vi "Add Virtual Instrument.vi"(8 "Error In":errorcluster, 9 "IVirtual Instrument":refnum<class "IVirtual Instrument.lvclass">, 10 "Instrument Identifier":string) -> (0 "Error Out":errorcluster)   [LabVIEW 2019, in "Instrument Manager.lvclass"]
uses:
  Instrument Manager.lvclass
  Instrument Manager.lvclass/Instrument Manager.ctl
  Interfaces/IVirtual Instrument/IVirtual Instrument.lvclass
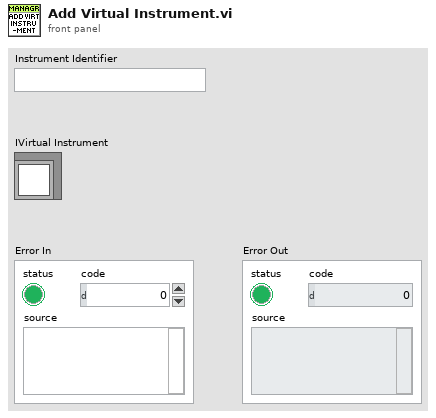
[diagram p1: front panel]
types:
  T1 = typedef "Instrument Manager.lvclass/ObjectAttributes.ctl" = cluster{"ICreate Action Point":refnum<class "ICreate Action Point.lvclass">, "IInstruments":map{string, refnum<class "IInstrument.lvclass">}, "IVirtual Instruments":map{string, refnum<class "IVirtual Instrument.lvclass">}, "Instrument Configurations":map{string, refnum<class "Config from JSON.lvclass">}, "Virtual Instrument Configurations":map{string, refnum<class "Config from JSON.lvclass">}, "Action Point Configurations":map{string, refnum<class "Config from JSON.lvclass">}, "Action Points":map{string, refnum<class "Action Point.lvclass">}}
  T2 = map{string, refnum<class "IVirtual Instrument.lvclass">}
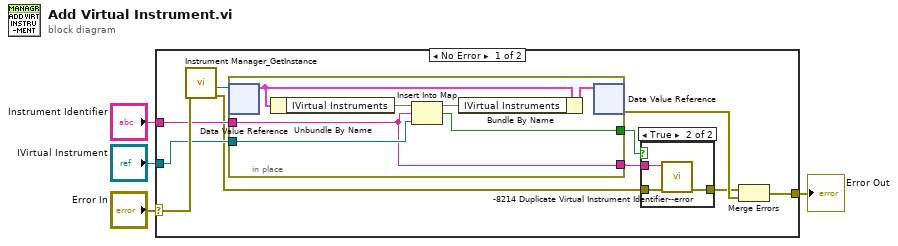
[diagram p0: block diagram]
diagram:
  n1 = case shown="No Error" "Error In" {
    selector: "Error In" -> [w14 w26]
    tunnel: [w12 w26] -> w3
    tunnel: "IVirtual Instrument" -> [w10 _]
    tunnel: "Instrument Identifier" -> [w9 _]
    frame No Error {
      n2 = call "Instrument Manager_GetInstance.vi"("Error In"=w14) -> ("Error Out"=w8:errorcluster, "DVRRefOut"=w11:refnum<data-value>)  [unwired: 6 in, 3 out]
      n3 = in-place {
        in-place-border: w10 -> [w21]
        in-place-border: w9 -> [w19]
        in-place-border: [w20] -> w6
        in-place-border: [w19] -> w5
        n4 = in-place-dvr #1(w11) -> (w24:T1)  [unwired: 1 out]
        n5 = Unbundle By Name(w24) -> ("IVirtual Instruments"=w23:T2)
        n6 = Insert Into Map(map in=w23, key=w19, value=w21) -> (map out=w22:T2, key already included?=w20:bool)  [unwired: 1 out]
        n7 = Bundle By Name(cluster=w24, "IVirtual Instruments"=w22) -> (w25:T1)
        n8 = in-place-dvr #1(w25) -> (w13:errorcluster)  [unwired: 1 out]
      }
      n9 = case shown="True" w6 {
        tunnel: w8 -> [w15 w18]
        tunnel: [w15 w17] -> w7
        tunnel: w5 -> [_ w16]
        frame False {
        }
        frame True {
          n10 = call "-8214 Duplicate Virtual Instrument Identifier--error.vi"("error in"=w18, "Virtual Instrument Identifier"=w16) -> ("error out"=w17:errorcluster)  [unwired: 9 in]
        }
      }
      n11 = Merge Errors(w7, w13) -> (w12:errorcluster)
    }
    frame Error {
    }
  }
  "Error Out" <- w3
